vi "W vs Z free space array.vi"(5 "FWHM(T)?":bool, 6 "Wavelength":dbl=0.0007 format="%.6f", 7 "Q start":cdb format="%.4f", 8 "N steps":i32=1, 9 "z stop":dbl=1000.0 format="%.2f", 10 "z start":dbl format="%.2f") -> (0 "Q out":cdb format="%.2f", 1 "Q Array":cxt[](array[numeric]) format="%.2f", 2 "w/FWHM Array":dbl[](array[numeric]) format="%.2f", 3 "Z Array":dbl[](array[numeric]) format="%.2f", 4 "W/FWHM vs Z":cluster{dbl[], dbl[]}(graph))   [LabVIEW 2012]
panel:
  out "sig min z":dbl format="%.2f"
  out "min signa w":dbl format="%.8f"
  in  "beam radius(w)":dbl=0.002 format="%.3f"
  in  "Radius of Curvature":dbl=inf format="%.2f"
  out "z step":dbl=1.0 format="%.3f"
  # "All values are entered in mm"
  # "w is the 1/e field radius"
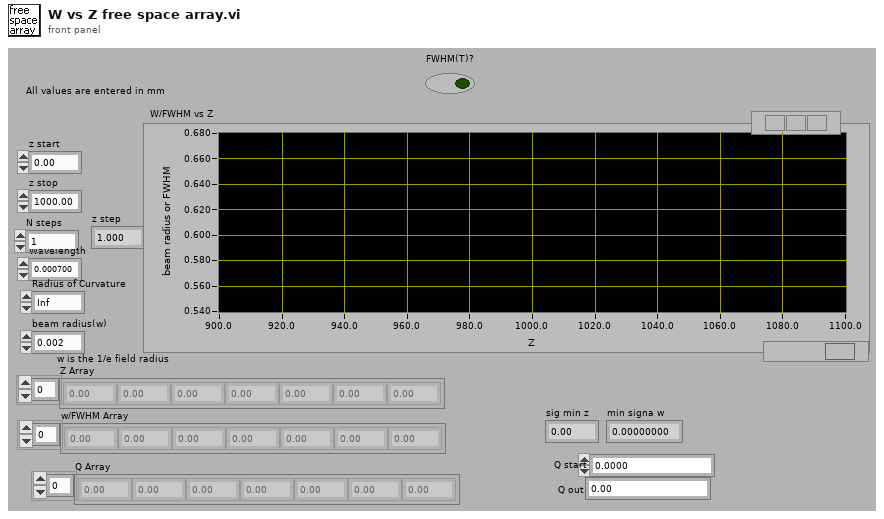
[diagram p1: front panel]
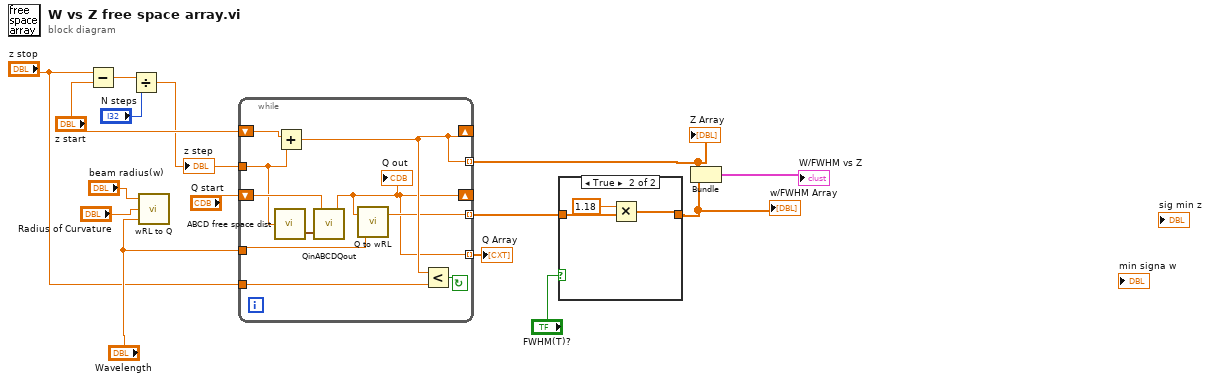
[diagram p0: block diagram]
diagram:
  n1 = Subtract(x="z stop", y="z start") -> (x-y=w10:dbl)
  n2 = Divide(x=w10, y="N steps") -> (x/y=w8:dbl)
  "z step" <- w8
  n3 = call "wRL to Q.vi"("Wavelength"="Wavelength", "Radius of Curvature"="Radius of Curvature", "beam radius(w)"="beam radius(w)") -> ()  [unwired: 1 out]
  n4 = while {
    shift-right: [w21] -> _
    shift-left: "z start" -> [w19]
    tunnel: w8 -> [w20]
    shift-right: [w16] -> _
    shift-left: "Q start" -> [w23]
    tunnel: "Wavelength" -> [w22]
    tunnel: [w17] -> w2 mode=indexing
    tunnel: [w21] -> w6 mode=indexing
    tunnel: "z stop" -> [w18]
    tunnel: [w16] -> w5 mode=indexing
    stop <- w25 continue-if-true
    n5 = call "ABCD free space dist.vi"("Dist"=w20) -> ("ABCD"=w24:cluster{"A":dbl, "B":dbl, "C":dbl, "D":dbl})
    n6 = Add(x=w19, y=w20) -> (x+y=w21:dbl)
    n7 = call "QinABCDQout.vi"("ABCD"=w24, "Q in"=w23) -> ("Q out"=w16:cdb)
    "Q out" <- w16
    n8 = call "Q to wRL.vi"("Wavelength"=w22, "Q"=w16) -> ("beam radius(w)"=w17:dbl)  [unwired: 1 out]
    n9 = Less?(x=w21, y=w18) -> (x < y?=w25:bool)
  }
  "Z Array" <- w6
  "Q Array" <- w5
  n10 = case shown="True" "FWHM(T)?" {
    tunnel: w2 -> [w26 w28]
    tunnel: [w26 w27] -> w1
    frame False {
    }
    frame True {
      n11 = Multiply(x=1.18, y=w28) -> (x*y=w27:dbl[])
    }
  }
  "w/FWHM Array" <- w1
  n12 = Bundle(w6, w1) -> (→"W/FWHM vs Z":cluster{dbl[], dbl[]})  [unwired: 1 in]
